vi "ReferenceCalibrationViRange.vi"(8 "error in":errorcluster) -> (0 "error out":errorcluster, 1 "vi reference":refnum<vi>, 2 "Labels":string[](array[string]), 3 "Ranges":refnum<vi>[](array[refnum]))   [LabVIEW 2016]
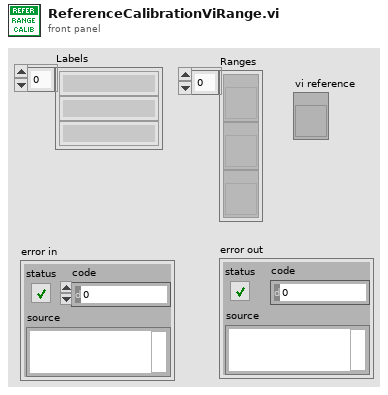
[diagram p1: front panel]
types:
  T1 = enum32{"Invalid", "Standard", "Closed", "Hidden", "Minimized", "Maximized"}
  T2 = enum32{"Bad", "Idle", "Run top level", "Running"}
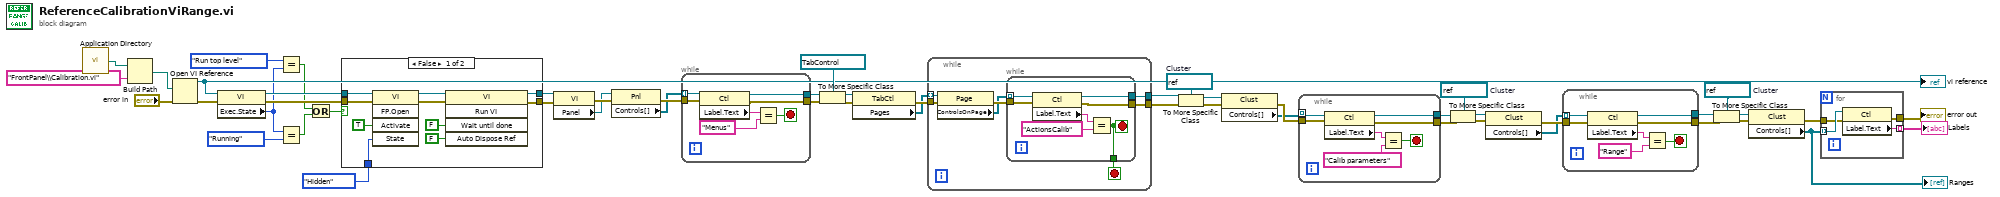
[diagram p0: block diagram]
diagram:
  w35 = refnum<vi> refnum  # Cluster
  w31 = refnum<vi> refnum  # Cluster
  w26 = refnum<vi> refnum  # Cluster
  n1 = call <vilib>:"Application Directory.vi"() -> ("Application Directory"=w18:path)
  n2 = Build Path(base path=w18, name or relative path="FrontPanel\\Calibration.vi") -> (appended path=w17:path)
  n3 = Open VI Reference(vi path=w17, error in (no error)="error in") -> (vi reference=w11:refnum<vi>, error out=w9:errorcluster)  [unwired: 4 in]
  "vi reference" <- w11
  n4 = property class="VI"(reference=w11, error in=w9) -> (reference out=w10:refnum<vi>, error out=w8:errorcluster, "Exec.State"=w3:T2)
  n5 = Equal?(x=T2."Run top level" ("Execution:State"), y=w3) -> (x = y?=w5:bool)
  n6 = Equal?(x=w3, y=T2."Running" ("Execution:State")) -> (x = y?=w4:bool)
  n7 = Or(x=w5, y=w4) -> (x .or. y?=w2:bool)
  n8 = case shown="False" w2 {
    tunnel: [w56 w62] -> w13
    tunnel: [w55 w63] -> w12
    tunnel: w10 -> [w54 w63]
    tunnel: w8 -> [w53 w62]
    tunnel: T1."Hidden" ("State") -> [w52 _]
    frame False {
      n9 = invoke class="VI" method="FP.Open"(reference=w54, error in=w53, "Activate"=TRUE ("Activate?"), "State"=w52) -> (reference out=w58:refnum<vi>, error out=w57:errorcluster)  [unwired: 1 in, 3 out]
      n10 = invoke class="VI" method="Run VI"(reference=w58, error in=w57, "Wait until done"=FALSE ("Wait Until Done"), "Auto Dispose Ref"=FALSE ("Auto Dispose Reference")) -> (reference out=w55:refnum<vi>, error out=w56:errorcluster)  [unwired: 1 in, 3 out]
    }
    frame True {
    }
  }
  n11 = property class="VI"(reference=w12, error in=w13) -> (error out=w50:errorcluster, "Panel"=w16:refnum<vi>)  [unwired: 1 out]
  n12 = property class="Pnl"(reference=w16, error in=w50) -> (error out=w51:errorcluster, "Controls[]"=w20:refnum<vi>[])  [unwired: 1 out]
  n13 = while {
    tunnel: w20 -> [w70] mode=indexing
    tunnel: [w67] -> w24
    tunnel: [w66] -> w49
    tunnel: w51 -> [w65]
    stop <- w68 stop-if-true
    n14 = property class="Ctl"(reference=w70, error in=w65) -> (reference out=w67:refnum<vi>, error out=w66:errorcluster, "Label.Text"=w64:string)
    n15 = Equal?(x=w64, y="Menus") -> (x = y?=w68:bool)
  }
  n16 = To More Specific Class(target class=refnum<vi> refnum ("Menus"), reference=w24, error in=w49) -> (specific class reference=w22:refnum<vi>, error out=w48:errorcluster)
  n17 = property class="TabCtl"(reference=w22, error in=w48) -> (error out=w47:errorcluster, "Pages"=w23:refnum<vi>[])  [unwired: 1 out]
  n18 = while {
    tunnel: w23 -> [w76] mode=indexing
    tunnel: [w73] -> w25
    tunnel: [w72] -> w46
    tunnel: w47 -> [w71]
    stop <- w74 stop-if-true
    n19 = property class="Page"(reference=w76, error in=w71) -> (error out=w77:errorcluster, "ControlsOnPage"=w75:refnum<vi>[])  [unwired: 1 out]
    n20 = while {
      tunnel: w75 -> [w84] mode=indexing
      tunnel: [w81] -> w74
      tunnel: [w80] -> w73
      tunnel: [w79] -> w72
      tunnel: w77 -> [w78]
      stop <- w81 stop-if-true
      n21 = property class="Ctl"(reference=w84, error in=w78) -> (reference out=w80:refnum<vi>, error out=w79:errorcluster, "Label.Text"=w83:string)
      n22 = Equal?(x=w83, y="ActionsCalib") -> (x = y?=w81:bool)
    }
  }
  n23 = To More Specific Class(target class=w26, reference=w25, error in=w46) -> (specific class reference=w27:refnum<vi>, error out=w28:errorcluster)
  n24 = property class="Clust"(reference=w27, error in=w28) -> (error out=w44:errorcluster, "Controls[]"=w29:refnum<vi>[])  [unwired: 1 out]
  n25 = while {
    tunnel: w29 -> [w91] mode=indexing
    tunnel: [w87] -> w30
    tunnel: w44 -> [w86]
    tunnel: [w85] -> w45
    stop <- w88 stop-if-true
    n26 = property class="Ctl"(reference=w91, error in=w86) -> (reference out=w87:refnum<vi>, error out=w85:errorcluster, "Label.Text"=w90:string)
    n27 = Equal?(x=w90, y="Calib parameters") -> (x = y?=w88:bool)
  }
  n28 = To More Specific Class(target class=w31, reference=w30, error in=w45) -> (specific class reference=w32:refnum<vi>, error out=w33:errorcluster)
  n29 = property class="Clust"(reference=w32, error in=w33) -> (error out=w42:errorcluster, "Controls[]"=w34:refnum<vi>[])  [unwired: 1 out]
  n30 = while {
    tunnel: w34 -> [w94] mode=indexing
    tunnel: [w95] -> w36
    tunnel: [w93] -> w41
    tunnel: w42 -> [w92]
    stop <- w96 stop-if-true
    n31 = property class="Ctl"(reference=w94, error in=w92) -> (reference out=w95:refnum<vi>, error out=w93:errorcluster, "Label.Text"=w98:string)
    n32 = Equal?(x=w98, y="Range") -> (x = y?=w96:bool)
  }
  n33 = To More Specific Class(target class=w35, reference=w36, error in=w41) -> (specific class reference=w37:refnum<vi>, error out=w38:errorcluster)
  n34 = property class="Clust"(reference=w37, error in=w38) -> (error out=w43:errorcluster, "Controls[]"=w39:refnum<vi>[])  [unwired: 1 out]
  "Ranges" <- w39
  n35 = for {
    tunnel: w39 -> [w102] mode=indexing
    tunnel: [w101] -> w40 mode=indexing
    tunnel: w43 -> [w100]
    tunnel: [w99] -> w15
    n36 = property class="Ctl"(reference=w102, error in=w100) -> (error out=w99:errorcluster, "Label.Text"=w101:string)  [unwired: 1 out]
  }
  "Labels" <- w40
  "error out" <- w15
